vi "Write Stop Module Loop.vi"(10 "Stop":bool, 11 "Module Ident":string) -> (2 "error out":errorcluster)   [LabVIEW 2024]
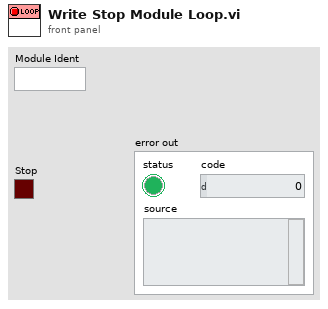
[diagram p1: front panel]
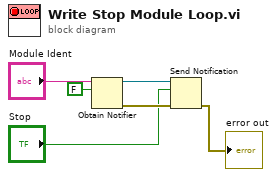
[diagram p0: block diagram]
diagram:
  n1 = Obtain Notifier(name (unnamed)="Module Ident", notification data type=FALSE) -> (notifier out=w4:refnum<notifier>, error out=w3:errorcluster)  [unwired: 2 in, 1 out]
  n2 = Send Notification(notification="Stop", notifier=w4, error in (no error)=w3) -> (error out=→"error out":errorcluster)  [unwired: 1 out]
